vi "Set Magnet.vi"(4 "Mode":T2, 6 "Axis":T1, 8 "error in (no error)":errorcluster, 9 "Target Rate (T/min)":dbl, 10 "Target Field (T)":dbl, 11 "instrument.PPMS":refnum<class "instrument.PPMS.lvclass">) -> (0 "error out":errorcluster, 3 "instrument.PPMS out":refnum<class "instrument.PPMS.lvclass">)   [LabVIEW 2019, in "instrument.PPMS.lvclass"]
uses:
  instrument.PPMS.lvclass
  C:/Program Files (x86)/National Instruments/LabVIEW 2019/user.lib/LevyLab/Instrument Framework/SMOs/Instrument/Instrument.lvclass
  <userlib>/LevyLab/Instrument Framework/Instrument Types/Cryostat/Typedefs/Magnet Mode--Enum.ctl
  <userlib>/LevyLab/Instrument Framework/Instrument Types/Cryostat/Typedefs/Magnet Axis--Enum.ctl
  <userlib>/LevyLab/Instrument Framework/Instrument Types/Cryostat/Typedefs/Set Magnet--cluster.ctl
  Typedefs/PPMS.Commands-enum.ctl
  <userlib>/LevyLab/Instrument Framework/SMOs/Instrument/Instrument.lvclass/Instrument.ctl
  eb731f9c-df04-47b0-80f7-775d271820e8.vi
  <vilib>/AdvancedString/1D String Array to Delimited String.vi
  eb731f9c-df04-47b0-80f7-775d271820e8.vi/2fda2d54-1ba6-4fda-9b62-b8739601108e.vi
  eb731f9c-df04-47b0-80f7-775d271820e8.vi/2fda2d54-1ba6-4fda-9b62-b8739601108e.vi/9c6c458e-3adf-40f4-a0ac-875b7f52f8d9.vi
  <userlib>/LevyLab/Instrument Framework/SMOs/Instrument/API/Send and Receive.vi
  eb731f9c-df04-47b0-80f7-775d271820e8.vi/2fda2d54-1ba6-4fda-9b62-b8739601108e.vi/14a0b3da-6916-4cef-a3e4-581aad1f6595.vi
  <userlib>/LevyLab/Instrument Framework/SMOs/Instrument/Private/Get Client Type.vi
  eb731f9c-df04-47b0-80f7-775d271820e8.vi/2fda2d54-1ba6-4fda-9b62-b8739601108e.vi/9c6c458e-3adf-40f4-a0ac-875b7f52f8d9.vi/a5a9d1dd-c463-4b6d-ba28-5ce4cd97edbd.vi
  eb731f9c-df04-47b0-80f7-775d271820e8.vi/2fda2d54-1ba6-4fda-9b62-b8739601108e.vi/9c6c458e-3adf-40f4-a0ac-875b7f52f8d9.vi/fda4e018-ffbe-4aa4-8f90-d559fc84fbfe.vi
  eb731f9c-df04-47b0-80f7-775d271820e8.vi/2fda2d54-1ba6-4fda-9b62-b8739601108e.vi/14a0b3da-6916-4cef-a3e4-581aad1f6595.vi/286e23c9-5705-4fe7-9793-93b145185ab5.vi
  eb731f9c-df04-47b0-80f7-775d271820e8.vi/2fda2d54-1ba6-4fda-9b62-b8739601108e.vi/14a0b3da-6916-4cef-a3e4-581aad1f6595.vi/606f8e95-486e-483e-b2c9-02e6f88d0b4b.vi
  eb731f9c-df04-47b0-80f7-775d271820e8.vi/2fda2d54-1ba6-4fda-9b62-b8739601108e.vi/14a0b3da-6916-4cef-a3e4-581aad1f6595.vi/286e23c9-5705-4fe7-9793-93b145185ab5.vi/a656a83d-2253-41b7-b850-0c3785f1ec97.vi
  eb731f9c-df04-47b0-80f7-775d271820e8.vi/2fda2d54-1ba6-4fda-9b62-b8739601108e.vi/14a0b3da-6916-4cef-a3e4-581aad1f6595.vi/286e23c9-5705-4fe7-9793-93b145185ab5.vi/cc5a8abc-62ef-48ed-8d2d-c0424ee87e3a.vi
  <userlib>/LevyLab/Instrument Framework/SMOs/Instrument/API/Enum to String.vi
  <userlib>/LevyLab/Instrument Framework/SMOs/Instrument/Private/Get RC Connection Status.vi
  <userlib>/LevyLab/Instrument Framework/SMOs/RemoteControl/API/Send and Receive.vi
  <vilib>/Utility/Data Type/Get Type Information.vi
  <vilib>/JDP Science/JSONtext/JSON text to Variant.vi
  <userlib>/LevyLab/Instrument Framework/SMOs/Instrument/API/Instrument.GetPublicEvents.vi
  <vilib>/JDP Science/JSONtext/Variant to JSON Text.vi
  <vilib>/National Instruments/GUID Generator/Guid Generator.vi
  <userlib>/LevyLab/Instrument Framework/SMOs/Instrument/API/Instrument.MessageToProcess.vi
  <userlib>/LevyLab/Instrument Framework/SMOs/Instrument/Private/Instrument.MessageFromProcess.EventStructure.vi
  <vilib>/Utility/error.llb/Error Cluster From Error Code.vi
  <vilib>/JDP Science/JSONtext/LVClass Serializer/JSONtext LVClass Serializer.lvclass
  <userlib>/LevyLab/Instrument Framework/Instrument Types/Cryostat/Instrument.Cryostat.lvclass
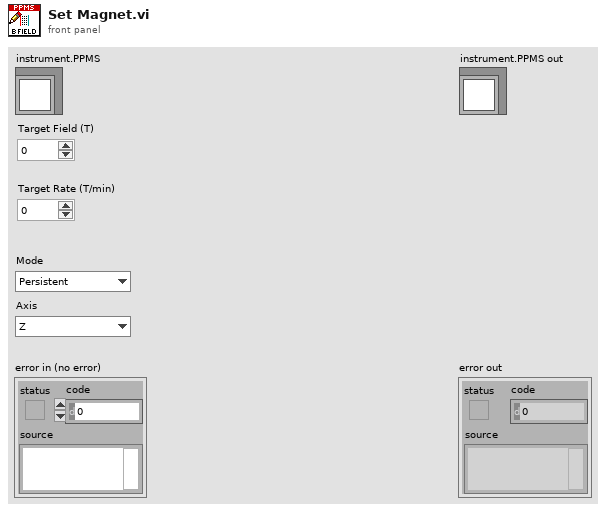
[diagram p1: front panel]
types:
  T1 = typedef "Instrument.Cryostat.lvclass/Magnet Axis--Enum.ctl" = enum16{"Z", "X", "Y"}
  T2 = typedef "Instrument.Cryostat.lvclass/Magnet Mode--Enum.ctl" = enum16{"Persistent", "Driven"}
  T3 = typedef "instrument.PPMS.lvclass/PPMS.Commands-enum.ctl" = enum16{"Get Angle", "Get Helium Level", "Get Magnet", "Get Temperature", "Set Angle", "Set Chamber", "Set Magnet", "Set Temperature", "getAll"}
  T4 = typedef "Instrument.Cryostat.lvclass/Set Magnet--cluster.ctl" = cluster{"Field (T)":dbl, "Rate (T/min)":dbl, "Axis":T1, "Mode":T2}
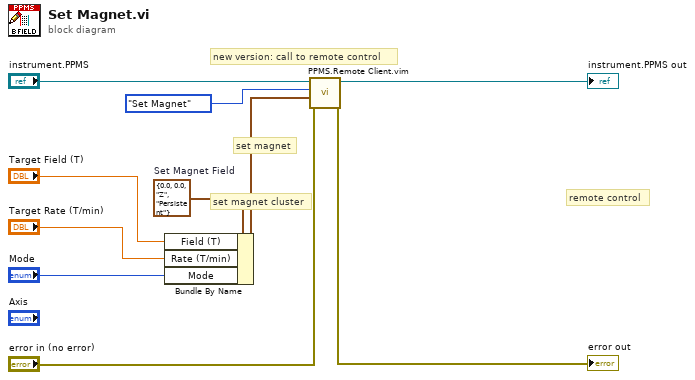
[diagram p0: block diagram]
diagram:
  w6 = T4 {"Field (T)"=0.0, "Rate (T/min)"=0.0, "Axis"=enum."Z", "Mode"=enum."Persistent"}  # Set Magnet Field
  # "set magnet cluster"
  # "remote control"
  # "set magnet"
  # "new version: call to remote control"
  n1 = Bundle By Name(cluster=w6, "Field (T)"="Target Field (T)", "Rate (T/min)"="Target Rate (T/min)", "Mode"="Mode") -> (w5:T4)
  n2 = call "PPMS.Remote Client.vim"("error in (no error)"="error in (no error)", "params"=w5, "Command"=PPMS.Commands-enum."Set Magnet", "instrument.PPMS in"="instrument.PPMS") -> ("error out"=→"error out":errorcluster, "instrument.PPMS out"=→"instrument.PPMS out":refnum<class "instrument.PPMS.lvclass">)  [unwired: 5 in, 1 out]
